vi "Add form.vi"(8 "error in (no error)":errorcluster, 9 "FK/PK Info":T1, 10 "Form ID":T2, 11 "Update Fields Logic Simple Table in":refnum<class "Update Fields Logic Simple Table.lvclass">) -> (0 "error out":errorcluster, 2 "Replaced?":bool, 3 "Update Fields Logic Simple Table out":refnum<class "Update Fields Logic Simple Table.lvclass">)   [LabVIEW 2020, in "Update Fields Logic Simple Table.lvlib" / "Update Fields Logic Simple Table.lvclass"]
uses:
  Update Fields Logic Simple Table.lvclass
  Autoclose manager/Form ID.ctl
  Update Fields Logic/Field FK PK Info.ctl
  Update Fields Logic Simple Table.lvclass/Update Fields Logic Simple Table.ctl
  Form Server Interfaces.lvlib
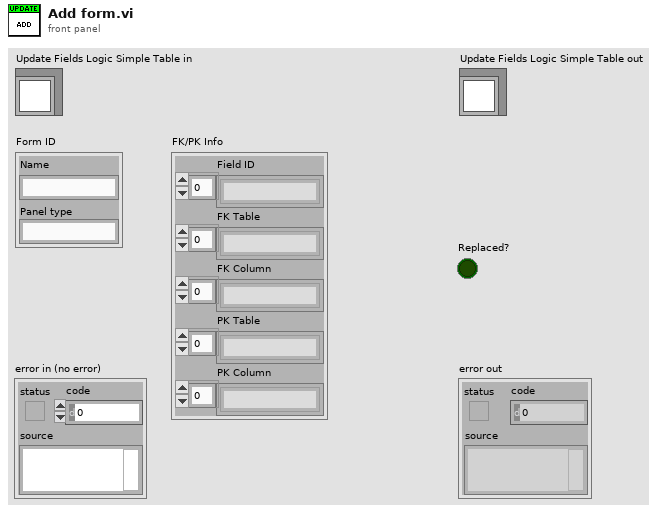
[diagram p1: front panel]
types:
  T1 = typedef "Form Server Interfaces.lvlib/Field FK PK Info.ctl" = cluster{"Field ID":string[], "FK Table":string[], "FK Column":string[], "PK Table":string[], "PK Column":string[]}
  T2 = typedef "Form Server Interfaces.lvlib/Form ID.ctl" = cluster{"Name":string, "Panel type":string}
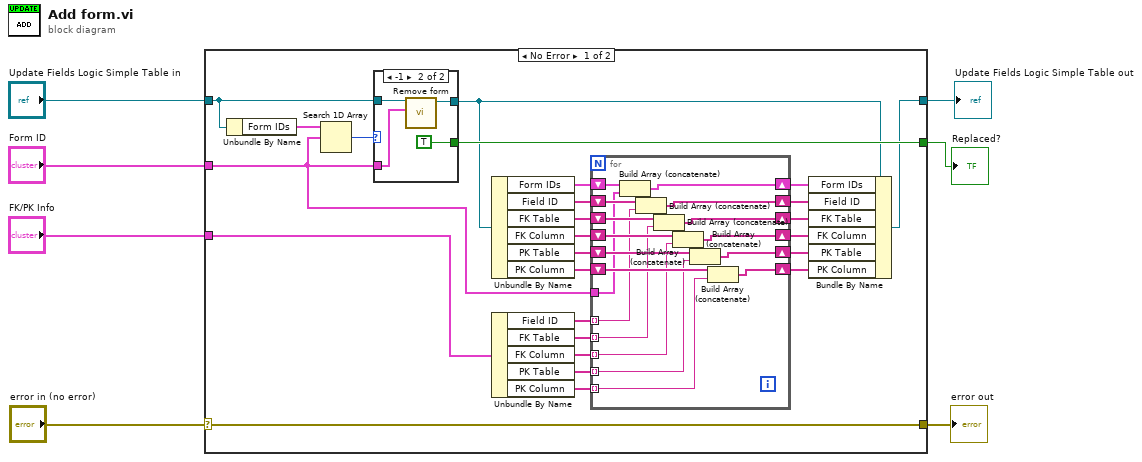
[diagram p0: block diagram]
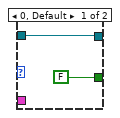
[diagram p2: hidden frame]
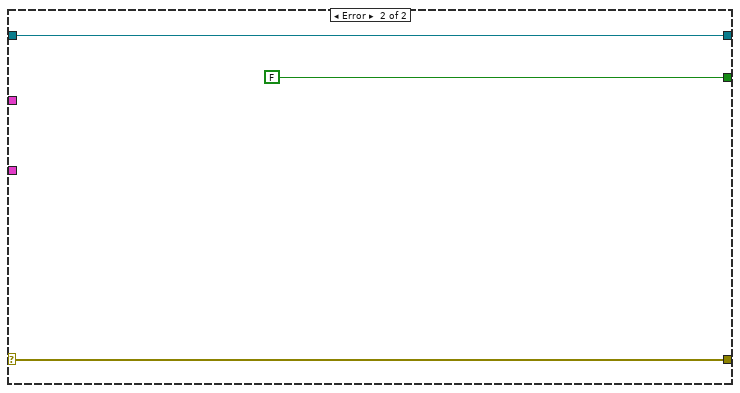
[diagram p3: hidden frame]
diagram:
  n1 = case shown="No Error" "error in (no error)" {
    selector: "error in (no error)" -> [w33 w59]
    tunnel: [w33 w59] -> w6
    tunnel: "Update Fields Logic Simple Table in" -> [w30 w60]
    tunnel: [w14 w60] -> w4
    tunnel: "Form ID" -> [w27 _]
    tunnel: "FK/PK Info" -> [w28 _]
    tunnel: [w29 FALSE] -> w1
    frame No Error {
      n2 = Unbundle By Name(w30) -> ("Form IDs"=w32:T2[])
      n3 = Search 1D Array(1D array=w32, element=w27) -> (index of element=w31:i32)  [unwired: 1 in]
      n4 = case shown="-1" w31 {
        tunnel: w30 -> [w53 w57]
        tunnel: [w53 w56] -> w15
        tunnel: w27 -> [_ w55]
        tunnel: [FALSE TRUE] -> w29
        frame 0, Default {
        }
        frame -1 {
          n5 = call-dynamic "Remove form.vi"("Form ID"=w55, "Update Fields Logic Simple Table in"=w57) -> ("Update Fields Logic Simple Table out"=w56:refnum<class "Update Fields Logic Simple Table.lvclass">)  [unwired: 8 in, 1 out]
        }
      }
      n6 = Unbundle By Name(w15) -> ("Form IDs"=w22:T2[], "Field ID"=w21:string[], "FK Table"=w20:string[], "FK Column"=w19:string[], "PK Table"=w18:string[], "PK Column"=w17:string[])
      n7 = Unbundle By Name(w28) -> ("Field ID"=w26:string[], "FK Table"=w25:string[], "FK Column"=w24:string[], "PK Table"=w23:string[], "PK Column"=w16:string[])
      n8 = for {
        tunnel: w27 -> [w39]
        tunnel: w26 -> [w38] mode=indexing
        tunnel: w25 -> [w37] mode=indexing
        tunnel: w24 -> [w36] mode=indexing
        tunnel: w23 -> [w35] mode=indexing
        shift-right: [w45] -> w13
        shift-left: w22 -> [w51]
        shift-right: [w44] -> w12
        shift-left: w21 -> [w50]
        shift-right: [w43] -> w11
        shift-left: w20 -> [w49]
        shift-right: [w42] -> w10
        shift-left: w19 -> [w48]
        shift-right: [w41] -> w9
        shift-left: w18 -> [w47]
        shift-right: [w40] -> w8
        shift-left: w17 -> [w46]
        tunnel: w16 -> [w34] mode=indexing
        n9 = Build Array (concatenate)(w51, w39) -> (w45:T2[])
        n10 = Build Array (concatenate)(w50, w38) -> (w44:string[])
        n11 = Build Array (concatenate)(w49, w37) -> (w43:string[])
        n12 = Build Array (concatenate)(w48, w36) -> (w42:string[])
        n13 = Build Array (concatenate)(w47, w35) -> (w41:string[])
        n14 = Build Array (concatenate)(w46, w34) -> (w40:string[])
      }
      n15 = Bundle By Name(cluster=w15, "Form IDs"=w13, "Field ID"=w12, "FK Table"=w11, "FK Column"=w10, "PK Table"=w9, "PK Column"=w8) -> (w14:refnum<class "Update Fields Logic Simple Table.lvclass">)
    }
    frame Error {
    }
  }
  "error out" <- w6
  "Update Fields Logic Simple Table out" <- w4
  "Replaced?" <- w1
